vi "Periodic Tasks.vi"(3 "error in":errorcluster) -> ()   [LabVIEW 2020]
doc: "This VI runs in parallel to other tasks. It can contain as many user-defined periodic loops as you need. These can carry out PID or other sorts of timed response."
uses:
  Robot Global Data.vi
  <vilib>/Rock Robotics/WPI/DriverStation/WPI_DriverStationRobotMode2.ctl
  mechanisms.ctl
  <vilib>/Rock Robotics/WPI/ThirdParty/Phoenix-LabVIEW/Motor Controller/Controls/CTRE_Phoenix_MotorControl_ControlMode.ctl
  <vilib>/Rock Robotics/WPI/Solenoid/WPI_SolenoidValue.ctl
  <vilib>/Rock Robotics/WPI/Solenoid/WPI_SolenoidSetEnum.vi
  <vilib>/Rock Robotics/WPI/Solenoid/Deprecated/WPI_SolenoidGetBool.vi
  <vilib>/Rock Robotics/WPI/ThirdParty/REV Robotics/REVLib/Typedef/Spark MAX Control Type.ctl
  <vilib>/Rock Robotics/Network Tables/NT Write Number.vi
  <vilib>/Rock Robotics/Network Tables/NT Write String.vi
  <vilib>/Rock Robotics/WPI/Compressor/WPI_CompressorFeedbackMode.ctl
  <vilib>/Rock Robotics/Network Tables/NT Write Numeric Array.vi
  <vilib>/Rock Robotics/WPI/DriverStation/WPI_DriverStationAllianceInfo.ctl
  <vilib>/Rock Robotics/WPI/Joystick/WPI_JoystickDeviceEnum.ctl
  <vilib>/Rock Robotics/WPI/Joystick/WPI_JoystickDevRef.ctl
  Front Left Output.ctl
  Back Left Outputctl.ctl
  Back Right Output.ctl
  Front Right Output.ctl
panel:
  in  "HIgh Left 2":dbl=-100.0
  in  "High Right 2":dbl=-100.0
  in  "Reset Position":bool
  in  "High Right":dbl=-100.0
  in  "Elevator Dealy":i32=80
  out "Left Pulse Switch":bool
  out "Right Pulse Switch":bool
  in  "HIgh Left":dbl=-100.0
  in  "Low Goal":dbl=10.0
  out "Back Right RPM":dbl
  out "Front Right RPM":dbl
  out "Back Left RPM":dbl
  out "Front Left RPM":dbl
  out "Alliance":T1
  in  "Align 90":bool
  out "Auto Step":dbl
  out "Front Left Drive Position":dbl
  out "Low Pressure":dbl
  in  "Piston Delay":i32=2
  out "Compressor Running":bool
  out "Enabled":bool
  in  "Disable Compressor":bool
  out "High Pressure":dbl(slide) scale=0.0..120.0
  in  "Max Pressure (PSI)":dbl(slide)=120.0 scale=0.0..120.0
  in  "Min Pressure (PSI)":dbl(slide)=100.0 scale=0.0..120.0
  out "Left Color":string
  out "Left Color":u32(colorbox)
  in  "Blue Calibration":cluster{"R":dbl, "G":dbl, "B":dbl}={"R"=0.159091, "G"=0.404537, "B"=0.435606}
  in  "Green Calibration":cluster{"R":dbl, "G":dbl, "B":dbl}={"R"=0.282, "G"=0.513, "B"=0.204}
  in  "Red Calibration":cluster{"R":dbl, "G":dbl, "B":dbl}={"R"=0.583685, "G"=0.333333, "B"=0.082982}
  in  "Yellow Calibration":cluster{"R":dbl, "G":dbl, "B":dbl}={"R"=0.309, "G"=0.524, "B"=0.166}
  in  "Rear Stop":dbl=-410.0
  in  "Front Stop":dbl=-280.0
  out "Right Color Match":string
  out "Right Color":u32(colorbox)
  out "Front Climber Switch":bool
  out "Rear Climber Switch":bool
  out "Claw Piston":bool
  out "Left Intake Piston":bool
  out "Right Intake Piston":bool
  out "Left Shooter":bool
  out "Right Shooter":bool
  out "Front Climber Postion":dbl
  out "Rear Climber Postion":dbl
  out "comp yaw":dbl=98.73633599999974 format="%#.1f"
  out "Linear Acceleration":T2={"LinearAcceleration X"=0.0, "LinearAcceleration Y"=0.002, "LinearAcceleration Z"=0.012}
  in  "Front Left Offset":dbl=589.0
  in  "Front Right Offset":dbl=547.0
  in  "Back Left Offset":dbl=743.0
  in  "Back Right Offset":dbl=1064.0
  out "Left Front Drive Output":T3={"Front Left Velocity"=-0.0, "Front Left Current Angle"=179.67273538762845, "Front Left Position (Raw Sensor Units)"=936}
  out "Back Left Drive Output":T4={"Back Left Back Velocity"=0.0, " Back Left Current Angle"=359.61772051724495, "Back Left Position (Raw Sensor Units)"=790}
  out "Back Right Drive Output":T5={"Back Right Velocity"=0.0, "Back Right Current Angle"=0.24094689976084283, "Back Left Position (Raw Sensor Units)"=126}
  out "Right  Front Drive Output":T6={"Front Right Velocity"=0.0, "Front Right Current Angle"=0.5093765258786789, "Front Right Position (Raw Sensor Units)"=548}
  in  "Joystick Addresses":cluster{"Auxillary":T7, "Driver":T7}
  # "Max RPM 5700"
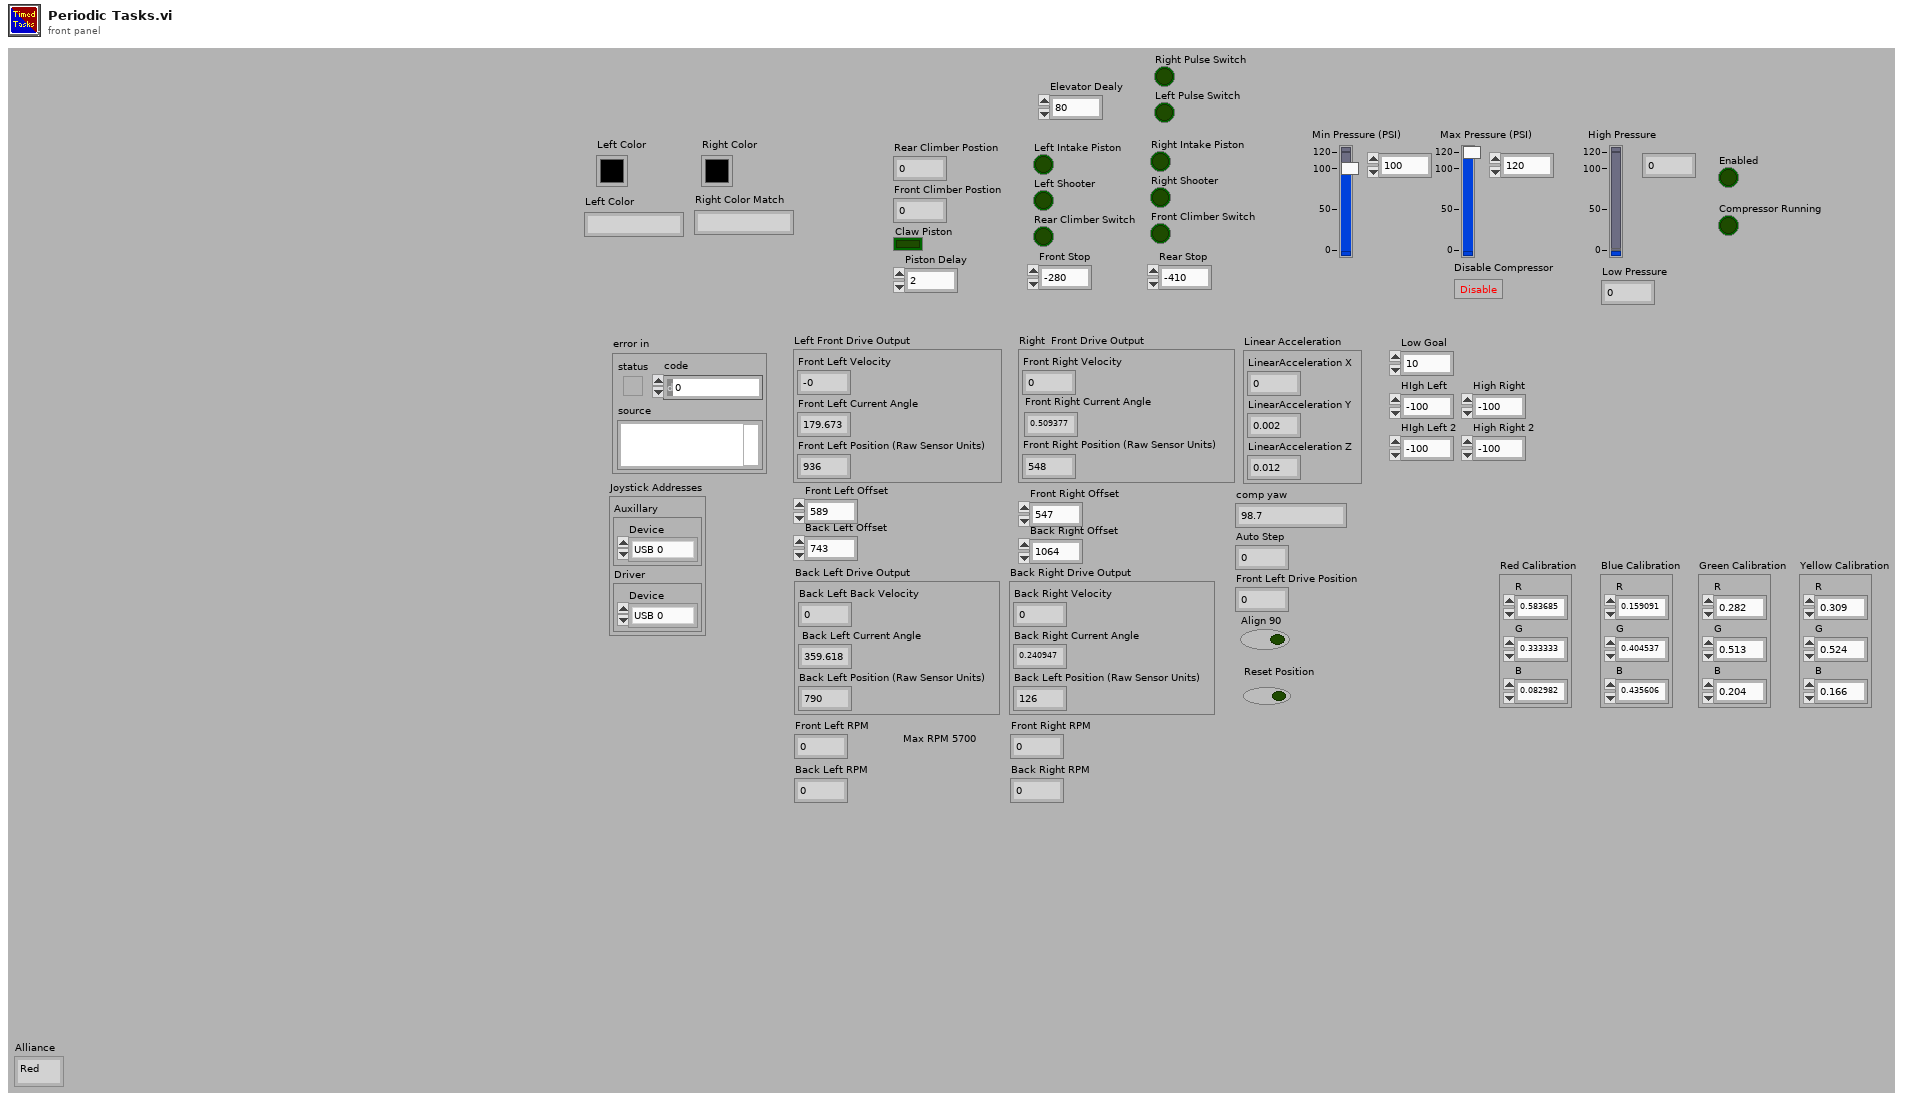
[diagram p1: front panel]
types:
  T1 = typedef "WPI_DriverStationAllianceInfo.ctl" = enum16{"Red", "Blue", "Invalid"}
  T2 = cluster{"LinearAcceleration X":dbl, "LinearAcceleration Y":dbl, "LinearAcceleration Z":dbl}
  T3 = typedef "Front Left Output.ctl" = cluster{"Front Left Velocity":dbl, "Front Left Current Angle":dbl, "Front Left Position (Raw Sensor Units)":i32}
  T4 = typedef "Back Left Outputctl.ctl" = cluster{"Back Left Back Velocity":dbl, " Back Left Current Angle":dbl, "Back Left Position (Raw Sensor Units)":i32}
  T5 = typedef "Back Right Output.ctl" = cluster{"Back Right Velocity":dbl, "Back Right Current Angle":dbl, "Back Left Position (Raw Sensor Units)":i32}
  T6 = typedef "Front Right Output.ctl" = cluster{"Front Right Velocity":dbl, "Front Right Current Angle":dbl, "Front Right Position (Raw Sensor Units)":i32}
  T7 = typedef "WPI_JoystickDevRef.ctl" = cluster{"Device":T8}
  T8 = typedef "WPI_JoystickDeviceEnum.ctl" = enum16{"USB 0", "USB 1", "USB 2", "USB 3", "USB 4", "USB 5"}
  T9 = typedef "WPI_DriverStationRobotMode2.ctl" = enum16{"Autonomous Disabled", "Autonomous Enabled", "Teleop Disabled", "Teleop Enabled", "Disconnected", "Finish", "Test Disabled", "Test Enabled", "Emergency Stopped"}
  T10 = typedef "mechanisms.ctl" = string
  T11 = cluster{"Yaw":dbl, "Roll":dbl, "Pitch":dbl, "Heading":dbl, "Fused Heading":dbl}
  T12 = cluster{"L X Axis":dbl, "L Y Axis":dbl, "LT":dbl, "RT":dbl, "R X Axis":dbl, "R Y Axis":dbl}
  T13 = cluster{"A":bool, "B":bool, "X":bool, "Y":bool, "LB":bool, "RB":bool, "Back":bool, "Start":bool, "Left Stick Push":bool, "Right Stick Push":bool}
  T14 = typedef "Color Sensor V3 DevRef.ctl" = cluster{"I2CDevRef":T15}
  T15 = typedef "WPI_I2CDevRef.ctl" = cluster{"DevStatus":errorcluster, "Device Address":u8, "Handle":i32, "I2C Bus":T16}
  T16 = typedef "i2c_bus.ctl" = enum16{"I2C On-Board", "I2C MXP", "Invalid"}
  T17 = typedef "WPI_MotorControlDeviceRef.ctl" = cluster{"DeviceStatus":errorcluster, "Type":T18, "PWM":cluster{"PWM Channel":T19, "DeadBand":T20}, "CAN":cluster{"Device Number":u8, "SetOutput VI Ref":variant, "GetOutput VI Ref":variant, "Enable VI Ref":variant, "Disable VI Ref":variant, "Data":variant}, "Invert":bool, "DIO PWM":cluster{"PWM \"Enable\" Channel":T19, "DIOChannel":T21, "PWM Rate":dbl}}
  T18 = typedef "WPI_MotorControlType.ctl" = enum16{"PWM", "CAN", "DIO PWM"}
  T19 = typedef "FPGA_DIOPWMChannel.ctl" = enum8{"PWM 0", "PWM 1", "PWM 2", "PWM 3", "PWM 4", "PWM 5", "PWM 6", "PWM 7", "PWM 8", "PWM 9", "PWM MXP 0", "PWM MXP 1", "PWM MXP 2", "PWM MXP 3", "PWM MXP 4", "PWM MXP 5", "PWM MXP 6", "PWM MXP 7", "PWM MXP 8", "PWM MXP 9", "Invalid"}
  T20 = typedef "WPI_PWMDeadband.ctl" = cluster{"Name":string, "maxPositivePwm":i32, "minPositivePwm":i32, "centerPwm":i32, "maxNegativePwm":i32, "minNegativePwm":i32, "angularRange":u16}
  T21 = typedef "FPGA_DIOChannel.ctl" = enum8{"DIO 0", "DIO 1", "DIO 2", "DIO 3", "DIO 4", "DIO 5", "DIO 6", "DIO 7", "DIO 8", "DIO 9", "DIO MXP 0", "DIO MXP 1", "DIO MXP 2", "DIO MXP 3", "DIO MXP 4", "DIO MXP 5", "DIO MXP 6", "DIO MXP 7", "DIO MXP 8", "DIO MXP 9", "DIO MXP 10", "DIO MXP 11", "DIO MXP 12", "DIO MXP 13", "DIO MXP 14", "DIO MXP 15", "SPI Port CS1", "SPI Port CS2", "SPI Port CS3", "SPI Port MISO", "SPI Port MOSI", "Invalid"}
  T22 = typedef "WPI_SolenoidValue.ctl" = enum16{"Off", "On", "Forward", "Reverse"}
  T23 = typedef "WPI_DigitalInputDevRef.ctl" = cluster{"DevStatus":errorcluster, "DIO Channel":T21}
  T24 = typedef "WPI_SolenoidDevRef.ctl" = cluster{"DevStatus":errorcluster, "Pneumatics Control Module":u8, "Forward Solenoid Channel":T25, "Reverse Solenoid Channel":T25}
  T25 = typedef "WPI_SolenoidChannel.ctl" = enum8{"Solenoid 0", "Solenoid 1", "Solenoid 2", "Solenoid 3", "Solenoid 4", "Solenoid 5", "Solenoid 6", "Solenoid 7", "Solenoid 8", "Solenoid 9", "Solenoid 10", "Solenoid 11", "Solenoid 12", "Solenoid 13", "Solenoid 14", "Solenoid 15", "Invalid"}
  T26 = typedef "CTRE_Phoenix_MotorControl_ControlMode.ctl" = u16
  T27 = typedef "WPI_CompressorFeedbackMode.ctl" = enum16{"Analog Only", "Digital Only", "Hybrid"}
  T28 = cluster{"Feedback Sensor":T27, "Max Pressure (PSI)":dbl, "Min Pressure (PSI)":dbl}
  T29 = typedef "WPI_CompressorDevRef.ctl" = cluster{"DevStatus":errorcluster, "Pneumatics Control Module":u8}
  T30 = cluster{"Pressure 0 (psi)":dbl, "Pressure 1 (psi)":dbl}
  T31 = typedef "Direction Commands.ctl" = cluster{"Lateral - X":dbl, "Longitudinal - Y":dbl, "Rotational - Z":dbl}
  T32 = typedef "Drive Comands.ctl" = cluster{"Align Steer Motors":bool, "Brake":bool, "Coast":bool, "Autonomous":bool}
  T33 = typedef "Spark MAX Control Type.ctl" = enum16{"Percent VBus", "Voltage", "Velocity", "Position", "Smart Motion", "Current", "Smart Velocity"}
  T34 = typedef "WPI_SwitchDevRef.ctl" = cluster{"DevStatus":errorcluster, "DIO Channel":T21, "CntIndex":T35, "Normally Closed":bool}
  T35 = typedef "FPGA_CounterCtrSystemIndex.ctl" = enum8{"Ctr 0", "Ctr 1", "Ctr 2", "Ctr 3", "Ctr 4", "Ctr 5", "Ctr 6", "Ctr 7", "Invalid"}
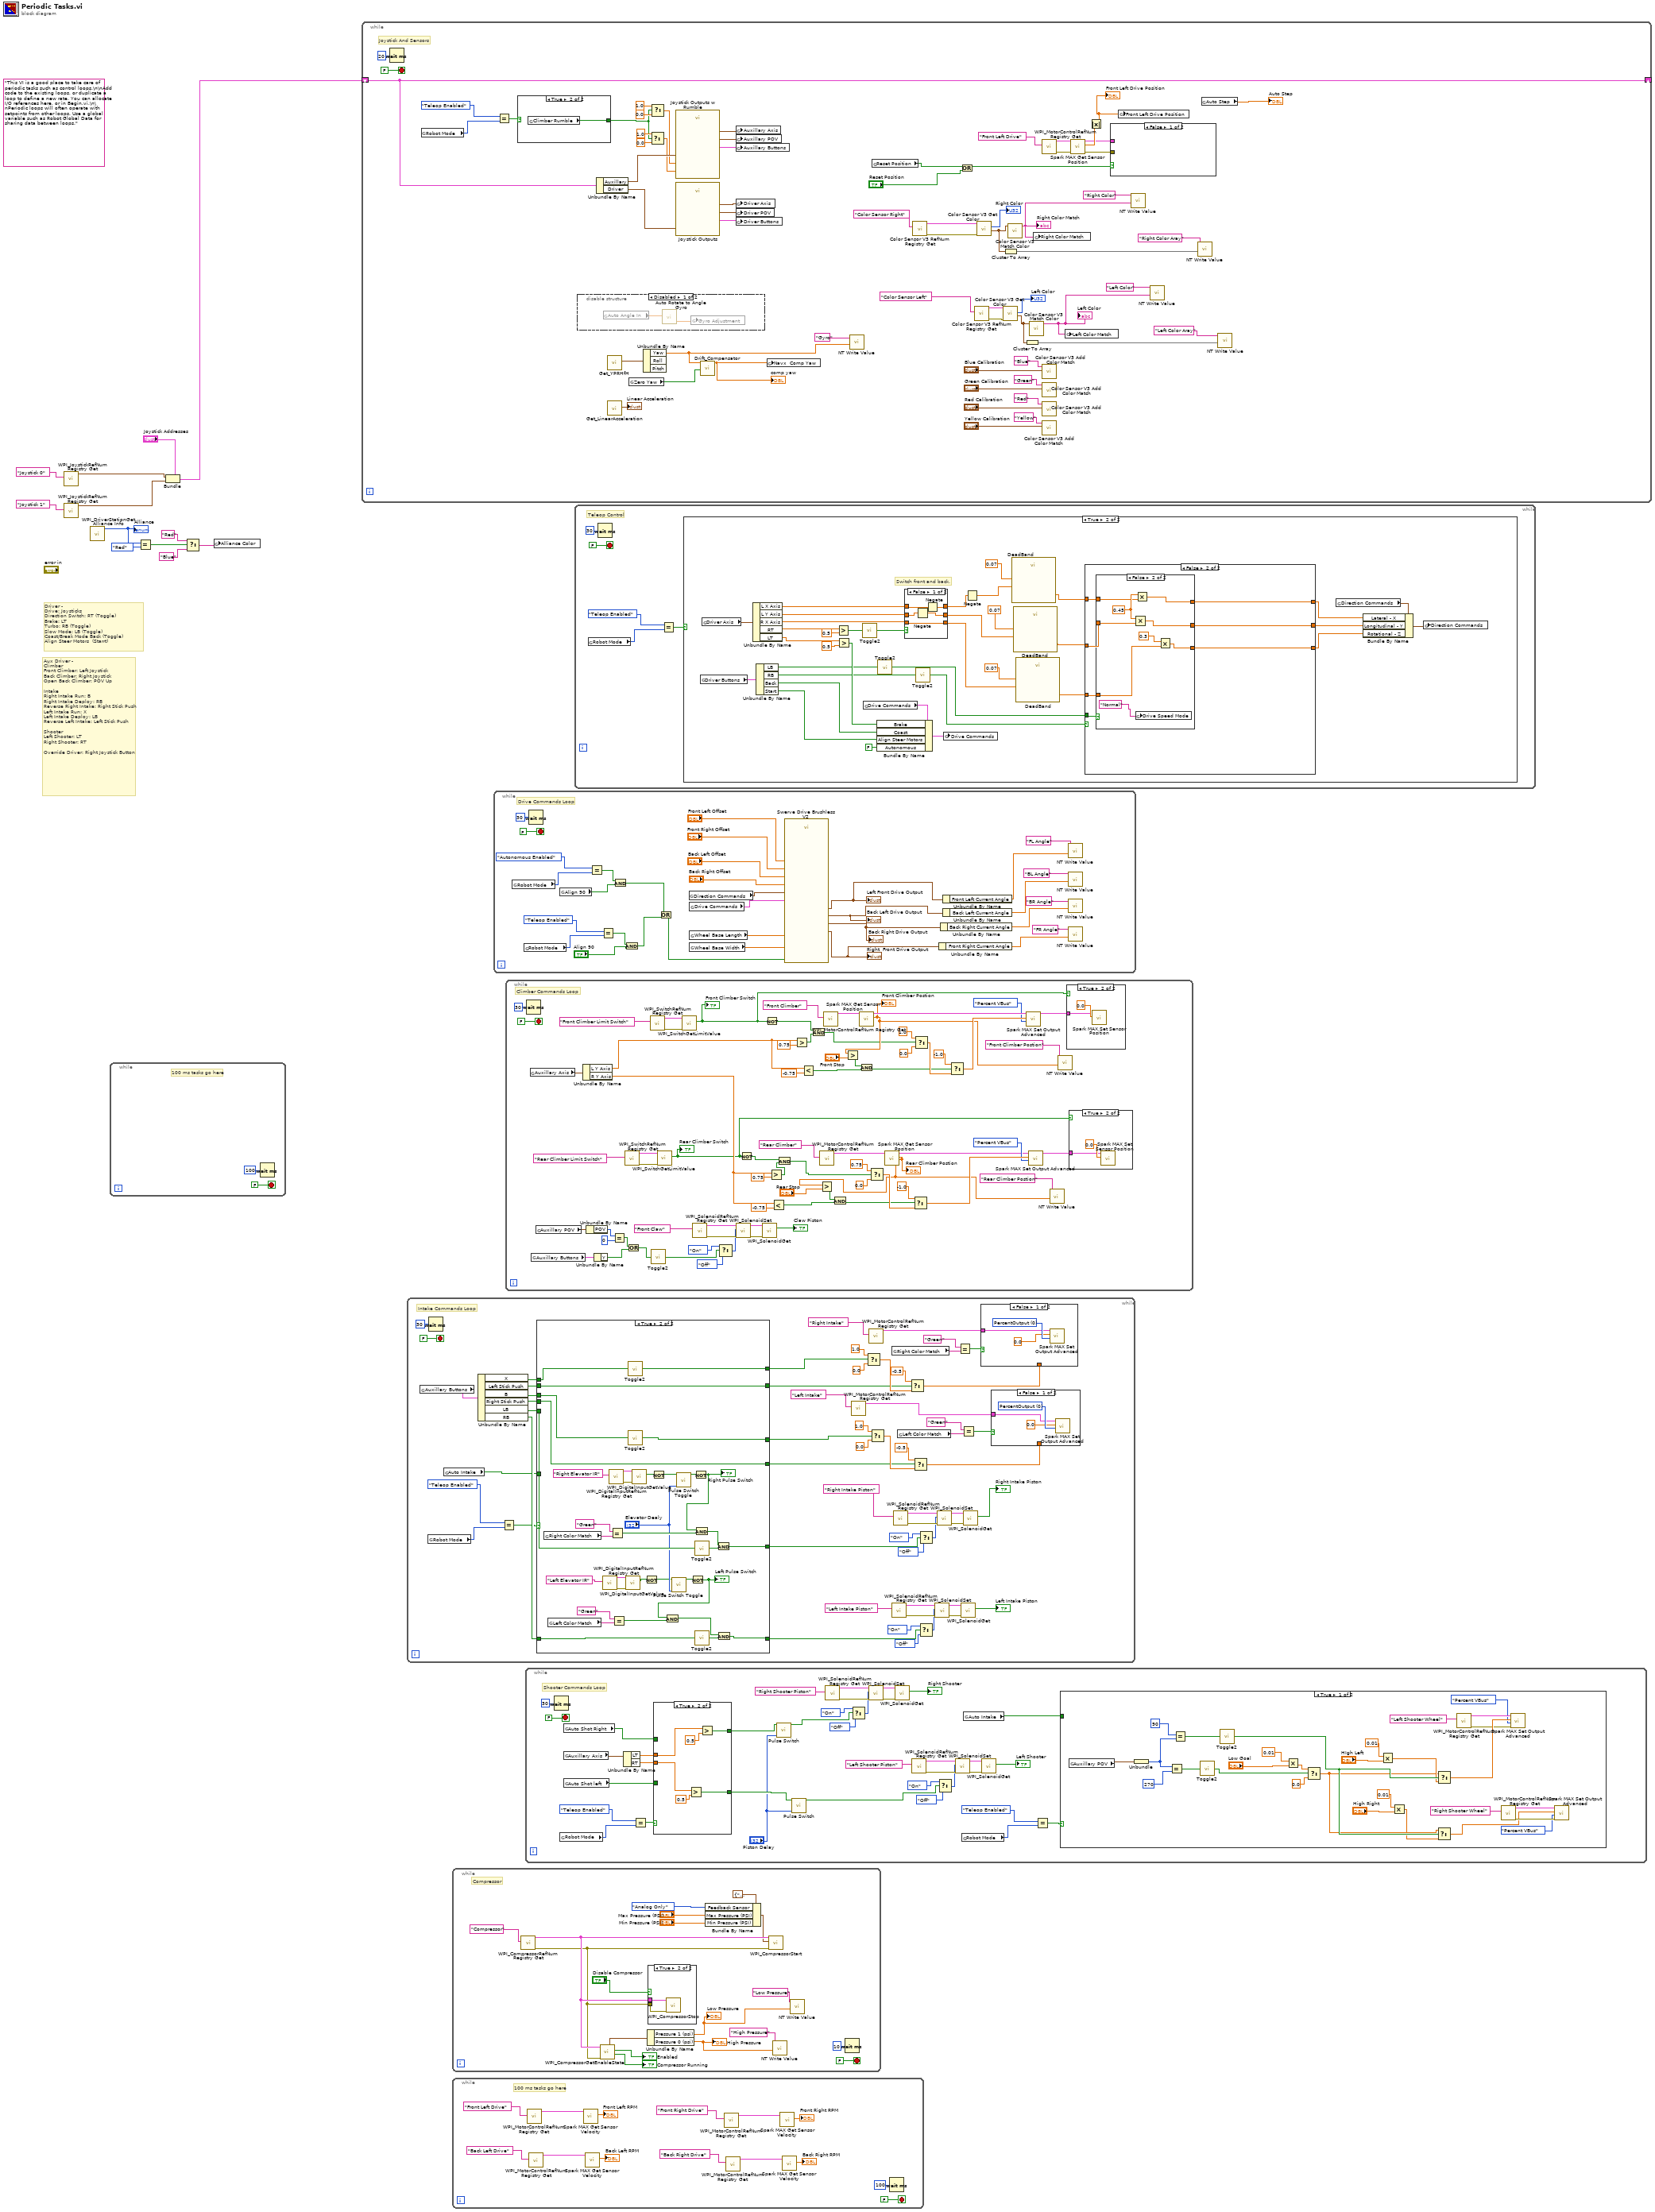
[diagram p0: block diagram]
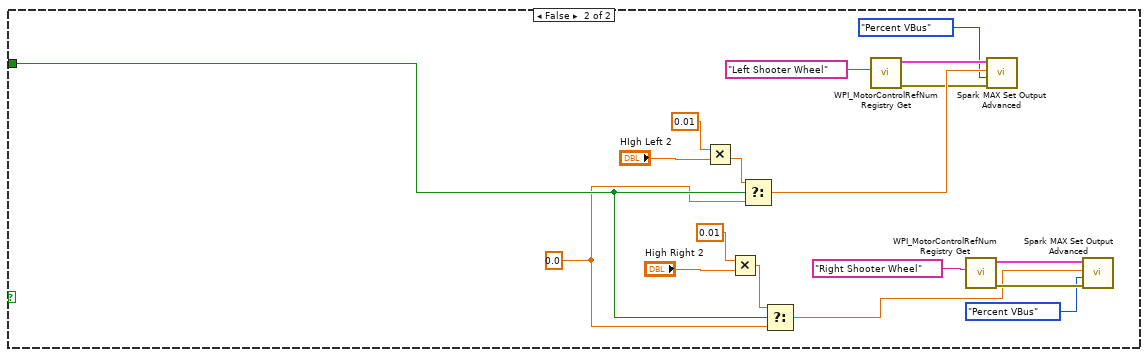
[diagram p3: hidden frame]
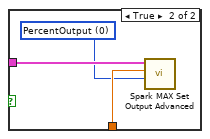
[diagram p5: hidden frame]
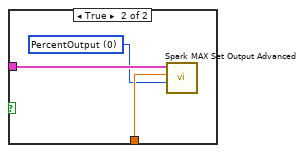
[diagram p6: hidden frame]
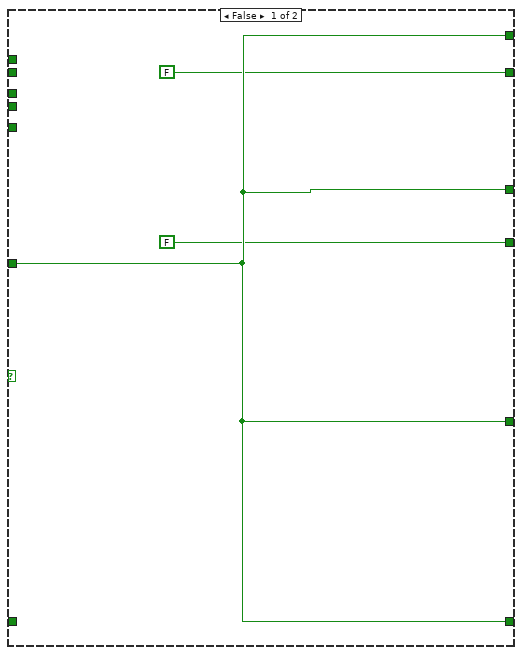
[diagram p7: hidden frame]
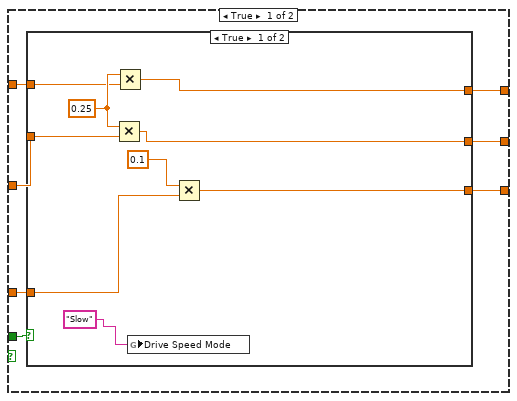
[diagram p11: hidden frame]
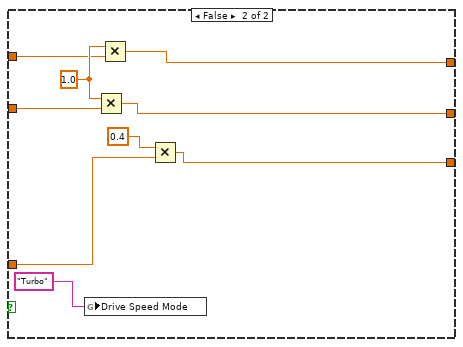
[diagram p12: hidden frame]
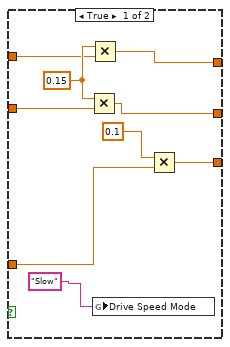
[diagram p13: hidden frame]
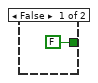
[diagram p15: hidden frame]
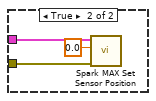
[diagram p17: hidden frame]
diagram:
  (unwired) "This VI is a good place to take care of periodic tasks such as control loops.\n\nAdd code to the existing loops, or duplicate a loop to define a new rate. You can allocate I/O references here, or in Begin.vi.\n\nPeriodic loops will often operate with setpoints from other loops. Use a global variable such as Robot Global Data for sharing data between loops."
  # "Aux Driver - \nClimber\nFront Climber: Left Joystick\nBack Climber: Right Joystick\nOpen Back Climber: POV Up\n\nIntake\nRight Intake Run: B\nRight Intake Deploy: RB\nReverse Right Intake: Right Stick Push\nLeft Intake Run: X\nLeft Intake Deploy: LB\nReverse Left Intake: Left Stick Push\n\nShooter\nLeft Shooter: LT\nRight Shooter: RT\n\nOverride Driver: Right Joystick Button"
  # "Driver - \nDrive: Joysticks\nDirection Switch: RT (Toggle)\nBrake: LT \nTurbo: RB (Toggle) \nSlow Mode: LB (Toggle) \nCoast/Break Mode Back (Toggle)\nAlign Steer Motors  (Starrt)"
  n1 = call <vilib>:"WPI_JoystickRefNum Registry Get.vi"("refnum name"="Joystick 0" ("Joystick Reference")) -> ("JoystickDevRef"=w10:T7)  [unwired: 9 in, 1 out]
  n2 = call <vilib>:"WPI_JoystickRefNum Registry Get.vi"("refnum name"="Joystick 1" ("Joystick Reference")) -> ("JoystickDevRef"=w9:T7)  [unwired: 9 in, 1 out]
  n3 = call <vilib>:"WPI_DriverStationGet Alliance Info.vi"() -> ("Alliance"=w6:T1)  [unwired: 6 in, 5 out]
  "Alliance" <- w6
  n4 = while {
    stop <- FALSE stop-if-true
    # "100 ms tasks go here"
    n5 = Wait (ms)(milliseconds to wait=u32 100) -> ()  [unwired: 1 out]
  }
  n6 = Equal?(x=w6, y=WPI_DriverStationAllianceInfo."Red") -> (x = y?=w4:bool)
  n7 = Bundle(cluster="Joystick Addresses", "Auxillary"=w10, "Driver"=w9) -> (w8:cluster{"Auxillary":T7, "Driver":T7})
  n8 = Select(t="Red" ("Right Color Match 2"), s=w4, f="Blue" ("Right Color Match 2")) -> (s? t:f=w1:string)
  n9 = global write "Robot Global Data.vi" "Alliance Color"(w1) -> ()
  n10 = while {
    shift-right: [w76] -> _
    shift-left: w8 -> [w76]
    stop <- FALSE stop-if-true
    # "Joystick And Sensors"
    n11 = Wait (ms)(milliseconds to wait=u32 20) -> ()  [unwired: 1 out]
    n12 = global read "Robot Global Data.vi" "Robot Mode"() -> (w17:T9)
    n13 = Equal?(x=WPI_DriverStationRobotMode2."Teleop Enabled", y=w17) -> (x = y?=w15:bool)
    n14 = case shown="True" w15 {
      tunnel: [FALSE ("Climber Rumble") w80] -> w20
      frame False {
      }
      frame True {
        n15 = global read "Robot Global Data.vi" "Climber Rumble"() -> (w80:bool)
      }
    }
    n16 = disable-structure shown="Disabled" {
      frame Disabled {
        n17 = global read "Robot Global Data.vi" "Auto Angle In"() -> (w82:dbl)
        n18 = call "Auto Rotate to Angle Gyro.vi"("Drive to Angle"=w82) -> ("Rotational Adjustment"=w81:dbl)  [unwired: 2 in]
        n19 = global write "Robot Global Data.vi" "Gyro Adjustment"(w81) -> ()
      }
      frame Enabled {
      }
    }
    n20 = Unbundle By Name(w76) -> ("Auxillary"=w75:T7, "Driver"=w74:T7)
    n21 = call <vilib>:"Get_YPRHfH.vi"() -> ("YRPHfH"=w63:T11)  [unwired: 11 in]
    n22 = call <vilib>:"Get_LinearAcceleration.vi"() -> ("Linear Acceleration"=→"Linear Acceleration":T2)  [unwired: 11 in]
    n23 = global read "Robot Global Data.vi" "Zero Yaw"() -> (w62:bool)
    n24 = Unbundle By Name(w63) -> ("Yaw"=w61:dbl)  [unwired: 2 out]
    n25 = Select(t=1.0, s=w20, f=0.0) -> (s? t:f=w23:dbl)
    n26 = Select(t=1.0, s=w20, f=0.0) -> (s? t:f=w28:dbl)
    n27 = call "Joystick Outputs w Rumble.vi"("Right Rumble"=w23, "Left Rumble"=w28, "JoystickDevRef"=w75) -> ("POV"=w72:cluster{"POV":i16}, "Axis"=w73:T12, "Buttons"=w71:T13)
    n28 = call "Joystick Outputs.vi"("JoystickDevRef"=w74) -> ("Buttons"=w68:T13, "Axis"=w70:T12, "POV"=w69:cluster{"POV":i16})
    n29 = call <vilib>:"Drift_Compensator.vi"("Zero Yaw"=w62, "Raw Yaw"=w61) -> ("comp yaw"=w60:dbl)  [unwired: 9 in]
    "comp yaw" <- w60
    n30 = global write "Robot Global Data.vi" "Auxillary Axis"(w73) -> ()
    n31 = global write "Robot Global Data.vi" "Auxillary POV"(w72) -> ()
    n32 = global write "Robot Global Data.vi" "Auxillary Buttons"(w71) -> ()
    n33 = global write "Robot Global Data.vi" "Driver Axis"(w70) -> ()
    n34 = global write "Robot Global Data.vi" "Driver POV"(w69) -> ()
    n35 = global write "Robot Global Data.vi" "Driver Buttons"(w68) -> ()
    n36 = global write "Robot Global Data.vi" "Navx  Comp Yaw"(w60) -> ()
    n37 = call-poly <vilib>:"NT Write Value.vi"("Numeric"=w61, "Name"="Gyro") -> ()  [unwired: 9 in, 1 out]
    n38 = global read "Robot Global Data.vi" "Reset Position"() -> (w31:bool)
    n39 = call <vilib>:"Color Sensor V3 RefNum Registry Get.vi"("refnum name"=T10 "Color Sensor Right" ("Mechanism")) -> ("error out"=w56:errorcluster, "ColorSensorDevRef"=w55:T14)  [unwired: 9 in]
    n40 = Or(x=w31, y="Reset Position") -> (x .or. y?=w19:bool)
    n41 = call <vilib>:"Color Sensor V3 RefNum Registry Get.vi"("refnum name"=T10 "Color Sensor Left" ("Mechanism")) -> ("error out"=w52:errorcluster, "ColorSensorDevRef"=w53:T14)  [unwired: 9 in]
    n42 = call <vilib>:"Color Sensor V3 Get Color.vi"("error in (no error)"=w56, "ColorSensorDevRef"=w55) -> ("Normalized Color"=w40:cluster{"R":dbl, "G":dbl, "B":dbl}, "Color"=→"Right Color":u32)  [unwired: 6 in, 2 out]
    n43 = call <vilib>:"Color Sensor V3 Get Color.vi"("error in (no error)"=w52, "ColorSensorDevRef"=w53) -> ("Normalized Color"=w36:cluster{"R":dbl, "G":dbl, "B":dbl}, "Color"=→"Left Color":u32)  [unwired: 6 in, 2 out]
    n44 = Cluster To Array(cluster=w40) -> (array=w39:dbl[])
    n45 = call <vilib>:"Color Sensor V3 Match Color.vi"("Measured Color"=w40) -> ("Matched Color Name"=w21:string)  [unwired: 8 in, 2 out]
    "Right Color Match" <- w21
    n46 = Cluster To Array(cluster=w36) -> (array=w35:dbl[])
    n47 = call <vilib>:"Color Sensor V3 Match Color.vi"("Measured Color"=w36) -> ("Matched Color Name"=w22:string)  [unwired: 8 in, 2 out]
    "Left Color" <- w22
    n48 = global write "Robot Global Data.vi" "Right Color Match"(w21) -> ()
    n49 = call <vilib>:"WPI_MotorControlRefNum Registry Get.vi"("refnum name"="Front Left Drive" ("Motor References")) -> ("error out"=w65:errorcluster, "RobotDriveDevRef"=w66:T17)  [unwired: 9 in]
    n50 = call <vilib>:"Color Sensor V3 Add Color Match.vi"("Color"="Blue Calibration", "Name"="Blue") -> ()  [unwired: 10 in]
    n51 = call <vilib>:"Color Sensor V3 Add Color Match.vi"("Color"="Green Calibration", "Name"="Green") -> ()  [unwired: 10 in]
    n52 = call <vilib>:"Color Sensor V3 Add Color Match.vi"("Color"="Red Calibration", "Name"="Red") -> ()  [unwired: 10 in]
    n53 = call <vilib>:"Color Sensor V3 Add Color Match.vi"("Color"="Yellow Calibration", "Name"="Yellow") -> ()  [unwired: 10 in]
    n54 = global write "Robot Global Data.vi" "Left Color Match"(w22) -> ()
    n55 = call <vilib>:"Spark MAX Get Sensor Position.vi"("error in (no error)"=w65, "MotorControlDevRef in"=w66) -> ("error out"=w32:errorcluster, "Sensor Position"=w34:dbl, "MotorControlDevRef out"=w33:T17)  [unwired: 6 in, 1 out]
    n56 = Absolute Value(x=w34) -> (abs(x)=w29:dbl)
    "Front Left Drive Position" <- w29
    n57 = case shown="False" w19 {
      tunnel: w33 -> [_ w85]
      tunnel: w32 -> [_ w84]
      frame False {
      }
      frame True {
        n58 = call <vilib>:"Spark MAX Set Sensor Position.vi"("error in"=w84, "Position"=0.0, "MotorControlDeviceRef"=w85) -> ()  [unwired: 7 in, 2 out]
      }
    }
    n59 = global write "Robot Global Data.vi" "Front Left Drive Position"(w29) -> ()
    n60 = call-poly <vilib>:"NT Write Value.vi"("String"=w21, "Name"="Right Color") -> ()  [unwired: 9 in, 1 out]
    n61 = call-poly <vilib>:"NT Write Value.vi"("String"=w22, "Name"="Left Color") -> ()  [unwired: 9 in, 1 out]
    n62 = call-poly <vilib>:"NT Write Value.vi"("Numeric Array"=w39, "Name"="Right Color Aray") -> ()  [unwired: 9 in, 1 out]
    n63 = global read "Robot Global Data.vi" "Auto Step"() -> (→"Auto Step":dbl)
    n64 = call-poly <vilib>:"NT Write Value.vi"("Numeric Array"=w35, "Name"="Left Color Aray") -> ()  [unwired: 9 in, 1 out]
  }
  n65 = while {
    stop <- FALSE stop-if-true
    # "Intake Commands Loop"
    n66 = global read "Robot Global Data.vi" "Auxillary Buttons"() -> (w140:T13)
    n67 = global read "Robot Global Data.vi" "Robot Mode"() -> (w99:T9)
    n68 = Wait (ms)(milliseconds to wait=u32 30) -> ()  [unwired: 1 out]
    n69 = global read "Robot Global Data.vi" "Auto Intake"() -> (w96:bool)
    n70 = Unbundle By Name(w140) -> ("X"=w124:bool, "Left Stick Push"=w93:bool, "B"=w125:bool, "Right Stick Push"=w91:bool, "LB"=w102:bool, "RB"=w101:bool)
    n71 = Equal?(x=WPI_DriverStationRobotMode2."Teleop Enabled", y=w99) -> (x = y?=w97:bool)
    n72 = case shown="True" w97 {
      tunnel: w125 -> [_ w192]
      tunnel: w124 -> [_ w191]
      tunnel: [w157 w190] -> w123
      tunnel: [w157 w180] -> w105
      tunnel: [w157 w177] -> w104
      tunnel: w102 -> [_ w189]
      tunnel: w101 -> [_ w188]
      tunnel: [w157 w187] -> w100
      tunnel: w96 -> [w157 _]
      tunnel: w93 -> [_ w186]
      tunnel: [FALSE ("Left Stick Push") w186] -> w92
      tunnel: w91 -> [_ w185]
      tunnel: [FALSE ("Right Stick Push") w185] -> w90
      frame False {
      }
      frame True {
        n73 = global read "Robot Global Data.vi" "Right Color Match"() -> (w183:string)
        n74 = global read "Robot Global Data.vi" "Left Color Match"() -> (w182:string)
        n75 = call <vilib>:"WPI_DigitalInputRefNum Registry Get.vi"("refnum name"=T10 "Left Elevator IR" ("Mechanisms")) -> ("error out"=w173:errorcluster, "DigitalInputDevRef"=w172:T23)  [unwired: 9 in]
        n76 = call <vilib>:"WPI_DigitalInputRefNum Registry Get.vi"("refnum name"=T10 "Right Elevator IR" ("Mechanisms")) -> ("error out"=w175:errorcluster, "DigitalInputDevRef"=w174:T23)  [unwired: 9 in]
        n77 = Equal?(x="Green", y=w183) -> (x = y?=w169:bool)
        n78 = Equal?(x="Green", y=w182) -> (x = y?=w167:bool)
        n79 = call <vilib>:"WPI_DigitalInputGetValue.vi"("error in (no error)"=w173, "DigitalInputDevRef"=w172) -> ("Value"=w170:bool)  [unwired: 7 in, 2 out]
        n80 = call "Toggle2.vi"("In 2"=w191) -> ("Out 2"=w187:bool)
        n81 = call "Toggle2.vi"("In 2"=w192) -> ("Out 2"=w190:bool)
        n82 = call <vilib>:"WPI_DigitalInputGetValue.vi"("error in (no error)"=w175, "DigitalInputDevRef"=w174) -> ("Value"=w166:bool)  [unwired: 7 in, 2 out]
        n83 = Not(x=w170) -> (.not. x?=w162:bool)
        n84 = Not(x=w166) -> (.not. x?=w163:bool)
        n85 = call "Pulse Switch Toggle.vi"("Input Switch"=w162, "Time/Loop Time"="Elevator Dealy") -> ("Pulse Switch"=w168:bool)  [unwired: 7 in, 1 out]
        n86 = call "Pulse Switch Toggle.vi"("Input Switch"=w163, "Time/Loop Time"="Elevator Dealy") -> ("Pulse Switch"=w165:bool)  [unwired: 7 in, 1 out]
        n87 = Not(x=w168) -> (.not. x?=w160:bool)
        "Left Pulse Switch" <- w160
        n88 = And(x=w160, y=w167) -> (x .and. y?=w161:bool)
        n89 = Not(x=w165) -> (.not. x?=w158:bool)
        "Right Pulse Switch" <- w158
        n90 = call "Toggle2.vi"("In 2"=w189) -> ("Out 2"=w179:bool)
        n91 = call "Toggle2.vi"("In 2"=w188) -> ("Out 2"=w178:bool)
        n92 = And(x=w158, y=w169) -> (x .and. y?=w159:bool)
        n93 = And(x=w159, y=w179) -> (x .and. y?=w180:bool)
        n94 = And(x=w161, y=w178) -> (x .and. y?=w177:bool)
      }
    }
    n95 = call <vilib>:"WPI_MotorControlRefNum Registry Get.vi"("refnum name"=T10 "Left Intake" ("Mechanism")) -> ("RobotDriveDevRef"=w133:T17)  [unwired: 9 in, 1 out]
    n96 = Select(t=1.0, s=w100, f=0.0) -> (s? t:f=w131:dbl)
    n97 = call <vilib>:"WPI_MotorControlRefNum Registry Get.vi"("refnum name"=T10 "Right Intake" ("Mechanism")) -> ("RobotDriveDevRef"=w126:T17)  [unwired: 9 in, 1 out]
    n98 = Select(t=1.0, s=w123, f=0.0) -> (s? t:f=w138:dbl)
    n99 = call <vilib>:"WPI_SolenoidRefNum Registry Get.vi"("refnum name"=T10 "Left Intake Piston" ("Mechanism")) -> ("error out"=w113:errorcluster, "SolenoidDevRef"=w112:T24)  [unwired: 9 in]
    n100 = global read "Robot Global Data.vi" "Right Color Match"() -> (w95:string)
    n101 = call <vilib>:"WPI_SolenoidRefNum Registry Get.vi"("refnum name"=T10 "Right Intake Piston" ("Mechanism")) -> ("error out"=w122:errorcluster, "SolenoidDevRef"=w121:T24)  [unwired: 9 in]
    n102 = global read "Robot Global Data.vi" "Left Color Match"() -> (w88:string)
    n103 = Select(t=-0.5, s=w92, f=w131) -> (s? t:f=w128:dbl)
    n104 = Select(t=-0.5, s=w90, f=w138) -> (s? t:f=w135:dbl)
    n105 = Select(t=WPI_SolenoidValue."On" ("Value"), s=w104, f=WPI_SolenoidValue."Off" ("Value")) -> (s? t:f=w109:T22)
    n106 = Select(t=WPI_SolenoidValue."On" ("Value"), s=w105, f=WPI_SolenoidValue."Off" ("Value")) -> (s? t:f=w118:T22)
    n107 = call-poly <vilib>:"WPI_SolenoidSet.vi"("error in (no error)"=w113, "Value"=w109, "SolenoidDevRef"=w112) -> ("error out"=w110:errorcluster, "SolenoidDevRef"=w111:T24)  [unwired: 7 in]
    n108 = call-poly <vilib>:"WPI_SolenoidSet.vi"("error in (no error)"=w122, "Value"=w118, "SolenoidDevRef"=w121) -> ("error out"=w119:errorcluster, "SolenoidDevRef"=w120:T24)  [unwired: 7 in]
    n109 = Equal?(x="Green", y=w95) -> (x = y?=w87:bool)
    n110 = call-poly <vilib>:"WPI_SolenoidGet.vi"("error in (no error)"=w110, "SolenoidDevRef"=w111) -> ("Value"=→"Left Intake Piston":bool)  [unwired: 7 in, 2 out]
    n111 = Equal?(x="Green", y=w88) -> (x = y?=w86:bool)
    n112 = call-poly <vilib>:"WPI_SolenoidGet.vi"("error in (no error)"=w119, "SolenoidDevRef"=w120) -> ("Value"=→"Right Intake Piston":bool)  [unwired: 7 in, 2 out]
    n113 = case shown="False" w87 {
      tunnel: w128 -> [_ w154]
      tunnel: w126 -> [w149 w153]
      frame False {
        w151 = T26 0 items=["PercentOutput"=0, "Position"=1, "Velocity"=2, "Current"=3, "Follower"=5, "MotionProfile"=6, "MotionMagic"=7, "MotionMagicArc"=8, "MotionProfileArc"=10, "Disabled"=15] ("Control Mode")
        n114 = call <vilib>:"Spark MAX Set Output Advanced.vi"("Control Mode"=w151, "Setpoint"=0.0, "MotorControlDevRef"=w149) -> ()  [unwired: 7 in, 2 out]
      }
      frame True {
        w152 = T26 0 items=["PercentOutput"=0, "Position"=1, "Velocity"=2, "Current"=3, "Follower"=5, "MotionProfile"=6, "MotionMagic"=7, "MotionMagicArc"=8, "MotionProfileArc"=10, "Disabled"=15] ("Control Mode")
        n115 = call <vilib>:"Spark MAX Set Output Advanced.vi"("Control Mode"=w152, "Setpoint"=w154, "MotorControlDevRef"=w153) -> ()  [unwired: 7 in, 2 out]
      }
    }
    n116 = case shown="False" w86 {
      tunnel: w135 -> [_ w148]
      tunnel: w133 -> [w143 w147]
      frame False {
        w145 = T26 0 items=["PercentOutput"=0, "Position"=1, "Velocity"=2, "Current"=3, "Follower"=5, "MotionProfile"=6, "MotionMagic"=7, "MotionMagicArc"=8, "MotionProfileArc"=10, "Disabled"=15] ("Control Mode")
        n117 = call <vilib>:"Spark MAX Set Output Advanced.vi"("Control Mode"=w145, "Setpoint"=0.0, "MotorControlDevRef"=w143) -> ()  [unwired: 7 in, 2 out]
      }
      frame True {
        w146 = T26 0 items=["PercentOutput"=0, "Position"=1, "Velocity"=2, "Current"=3, "Follower"=5, "MotionProfile"=6, "MotionMagic"=7, "MotionMagicArc"=8, "MotionProfileArc"=10, "Disabled"=15] ("Control Mode")
        n118 = call <vilib>:"Spark MAX Set Output Advanced.vi"("Control Mode"=w146, "Setpoint"=w148, "MotorControlDevRef"=w147) -> ()  [unwired: 7 in, 2 out]
      }
    }
  }
  n119 = while {
    stop <- FALSE stop-if-true
    # "Compressor"
    n120 = call <vilib>:"WPI_CompressorRefNum Registry Get.vi"("refnum name"="Compressor") -> ("error out"=w201:errorcluster, "CompressorDevRef"=w202:T29)  [unwired: 9 in]
    n121 = call <vilib>:"WPI_CompressorGetEnableState.vi"("error in (no error)"=w201, "CompressorDevRef"=w202) -> ("Compressor Running"=→"Compressor Running":bool, "Enabled"=→"Enabled":bool, "Pressure Sensors"=w206:T30)  [unwired: 3 in, 4 out]
    n122 = Unbundle By Name(w206) -> ("Pressure 1 (psi)"=w193:dbl, "Pressure 0 (psi)"=w200:dbl)
    "High Pressure" <- w200
    "Low Pressure" <- w193
    n123 = case shown="True" "Disable Compressor" {
      tunnel: w201 -> [_ w212]
      tunnel: w202 -> [_ w211]
      frame False {
      }
      frame True {
        n124 = call <vilib>:"WPI_CompressorStop.vi"("error in (no error)"=w212, "CompressorDevRef"=w211) -> ()  [unwired: 8 in, 2 out]
      }
    }
    n125 = Bundle By Name(cluster=T28 {"Feedback Sensor"=enum."Digital Only", "Max Pressure (PSI)"=0.0, "Min Pressure (PSI)"=0.0} ("Feedback Configuration"), "Feedback Sensor"=WPI_CompressorFeedbackMode."Analog Only", "Max Pressure (PSI)"="Max Pressure (PSI)", "Min Pressure (PSI)"="Min Pressure (PSI)") -> (w197:T28)
    n126 = call <vilib>:"WPI_CompressorStart.vi"("error in (no error)"=w201, "Feedback Configuration"=w197, "CompressorDevRef"=w202) -> ()  [unwired: 7 in, 2 out]
    n127 = call-poly <vilib>:"NT Write Value.vi"("Numeric"=w200, "Name"="High Pressure") -> ()  [unwired: 9 in, 1 out]
    n128 = call-poly <vilib>:"NT Write Value.vi"("Numeric"=w193, "Name"="Low Pressure") -> ()  [unwired: 9 in, 1 out]
    n129 = Wait (ms)(milliseconds to wait=u32 10) -> ()  [unwired: 1 out]
  }
  n130 = while {
    stop <- FALSE stop-if-true
    # "100 ms tasks go here"
    n131 = call <vilib>:"WPI_MotorControlRefNum Registry Get.vi"("refnum name"="Front Left Drive" ("Motor References")) -> ("RobotDriveDevRef"=w224:T17)  [unwired: 9 in, 1 out]
    n132 = call <vilib>:"WPI_MotorControlRefNum Registry Get.vi"("refnum name"="Back Left Drive" ("Motor References")) -> ("RobotDriveDevRef"=w221:T17)  [unwired: 9 in, 1 out]
    n133 = call <vilib>:"Spark MAX Get Sensor Velocity.vi"("MotorControlDevRef in"=w224) -> ("Sensor Velocity"=→"Front Left RPM":dbl)  [unwired: 7 in, 3 out]
    n134 = call <vilib>:"Spark MAX Get Sensor Velocity.vi"("MotorControlDevRef in"=w221) -> ("Sensor Velocity"=→"Back Left RPM":dbl)  [unwired: 7 in, 3 out]
    n135 = call <vilib>:"WPI_MotorControlRefNum Registry Get.vi"("refnum name"="Front Right Drive" ("Motor References")) -> ("RobotDriveDevRef"=w218:T17)  [unwired: 9 in, 1 out]
    n136 = call <vilib>:"WPI_MotorControlRefNum Registry Get.vi"("refnum name"="Back Right Drive" ("Motor References")) -> ("RobotDriveDevRef"=w215:T17)  [unwired: 9 in, 1 out]
    n137 = call <vilib>:"Spark MAX Get Sensor Velocity.vi"("MotorControlDevRef in"=w218) -> ("Sensor Velocity"=→"Front Right RPM":dbl)  [unwired: 7 in, 3 out]
    n138 = call <vilib>:"Spark MAX Get Sensor Velocity.vi"("MotorControlDevRef in"=w215) -> ("Sensor Velocity"=→"Back Right RPM":dbl)  [unwired: 7 in, 3 out]
    n139 = Wait (ms)(milliseconds to wait=u32 100) -> ()  [unwired: 1 out]
  }
  n140 = while {
    stop <- FALSE stop-if-true
    # "Drive Commands Loop"
    n141 = global read "Robot Global Data.vi" "Robot Mode"() -> (w249:T9)
    n142 = global read "Robot Global Data.vi" "Robot Mode"() -> (w232:T9)
    n143 = Wait (ms)(milliseconds to wait=u32 30) -> ()  [unwired: 1 out]
    n144 = global read "Robot Global Data.vi" "Align 90"() -> (w246:bool)
    n145 = Equal?(x=WPI_DriverStationRobotMode2."Autonomous Enabled", y=w249) -> (x = y?=w247:bool)
    n146 = Equal?(x=WPI_DriverStationRobotMode2."Teleop Enabled", y=w232) -> (x = y?=w231:bool)
    n147 = And(x=w247, y=w246) -> (x .and. y?=w245:bool)
    n148 = And(x=w231, y="Align 90") -> (x .and. y?=w227:bool)
    n149 = Or(x=w245, y=w227) -> (x .or. y?=w228:bool)
    n150 = global read "Robot Global Data.vi" "Direction Commands"() -> (w252:T31)
    n151 = global read "Robot Global Data.vi" "Drive Commands"() -> (w253:T32)
    n152 = global read "Robot Global Data.vi" "Wheel Base Length"() -> (w251:dbl)
    n153 = global read "Robot Global Data.vi" "Wheel Base Width"() -> (w250:dbl)
    n154 = call <vilib>:"Swerve Drive Brushless V2.vi"("Front Left Offset"="Front Left Offset", "Direction"=w252, "Front Right Offset"="Front Right Offset", "Align 90"=w228, "Back Left  Offset"="Back Left Offset", "Wheel Base Length"=w251, "Back Right Offset"="Back Right Offset", "Drive Commands"=w253, "Wheel Base Width"=w250) -> ("Front Left Drive Output"=w244:T3, "Front Right Drive Output"=w241:T6, "Back Left Drive Output"=w243:T4, "Back Right Drive Output"=w242:T5)  [unwired: 3 in]
    "Left Front Drive Output" <- w244
    "Back Left Drive Output" <- w243
    "Back Right Drive Output" <- w242
    "Right  Front Drive Output" <- w241
    n155 = Unbundle By Name(w241) -> ("Front Right Current Angle"=w240:dbl)
    n156 = Unbundle By Name(w242) -> ("Back Right Current Angle"=w239:dbl)
    n157 = Unbundle By Name(w244) -> ("Front Left Current Angle"=w237:dbl)
    n158 = Unbundle By Name(w243) -> ("Back Left Current Angle"=w238:dbl)
    n159 = call-poly <vilib>:"NT Write Value.vi"("Numeric"=w237, "Name"="FL Angle") -> ()  [unwired: 9 in, 1 out]
    n160 = call-poly <vilib>:"NT Write Value.vi"("Numeric"=w238, "Name"="BL Angle") -> ()  [unwired: 9 in, 1 out]
    n161 = call-poly <vilib>:"NT Write Value.vi"("Numeric"=w239, "Name"="BR Angle") -> ()  [unwired: 9 in, 1 out]
    n162 = call-poly <vilib>:"NT Write Value.vi"("Numeric"=w240, "Name"="FR Angle") -> ()  [unwired: 9 in, 1 out]
  }
  n163 = while {
    stop <- FALSE stop-if-true
    # "Climber Commands Loop"
    n164 = Wait (ms)(milliseconds to wait=u32 30) -> ()  [unwired: 1 out]
    n165 = global read "Robot Global Data.vi" "Auxillary Axis"() -> (w329:T12)
    n166 = global read "Robot Global Data.vi" "Auxillary Buttons"() -> (w272:T13)
    n167 = global read "Robot Global Data.vi" "Auxillary POV"() -> (w271:cluster{"POV":i16})
    n168 = Unbundle By Name(w329) -> ("L Y Axis"=w303:dbl, "R Y Axis"=w298:dbl)
    n169 = Unbundle By Name(w271) -> ("POV"=w270:i16)
    n170 = Unbundle By Name(w272) -> ("Y"=w267:bool)
    n171 = Equal?(x=w270, y=i16 0) -> (x = y?=w268:bool)
    n172 = call <vilib>:"WPI_SwitchRefNum Registry Get.vi"("refnum name"=T10 "Rear Climber Limit Switch" ("Mechanisms")) -> ("error out"=w290:errorcluster, "SwitchDevRef"=w291:T34)  [unwired: 9 in]
    n173 = Or(x=w268, y=w267) -> (x .or. y?=w266:bool)
    n174 = call <vilib>:"WPI_SwitchRefNum Registry Get.vi"("refnum name"=T10 "Front Climber Limit Switch" ("Mechanisms")) -> ("error out"=w293:errorcluster, "SwitchDevRef"=w292:T34)  [unwired: 9 in]
    n175 = call "Toggle2.vi"("In 2"=w266) -> ("Out 2"=w306:bool)
    n176 = call <vilib>:"WPI_SwitchGetLimitValue.vi"("error in (no error)"=w290, "SwitchDevRef"=w291) -> ("Switch Pressed"=w286:bool)  [unwired: 7 in, 2 out]
    "Rear Climber Switch" <- w286
    n177 = call <vilib>:"WPI_SwitchGetLimitValue.vi"("error in (no error)"=w293, "SwitchDevRef"=w292) -> ("Switch Pressed"=w285:bool)  [unwired: 7 in, 2 out]
    "Front Climber Switch" <- w285
    n178 = call <vilib>:"WPI_SolenoidRefNum Registry Get.vi"("refnum name"=T10 "Front Claw" ("Mechanism")) -> ("error out"=w313:errorcluster, "SolenoidDevRef"=w312:T24)  [unwired: 9 in]
    n179 = Select(t=WPI_SolenoidValue."On" ("Value"), s=w306, f=WPI_SolenoidValue."Off" ("Value")) -> (s? t:f=w309:T22)
    n180 = call-poly <vilib>:"WPI_SolenoidSet.vi"("error in (no error)"=w313, "Value"=w309, "SolenoidDevRef"=w312) -> ("error out"=w310:errorcluster, "SolenoidDevRef"=w311:T24)  [unwired: 7 in]
    n181 = Not(x=w286) -> (.not. x?=w262:bool)
    n182 = call-poly <vilib>:"WPI_SolenoidGet.vi"("error in (no error)"=w310, "SolenoidDevRef"=w311) -> ("Value"=→"Claw Piston":bool)  [unwired: 7 in, 2 out]
    n183 = Not(x=w285) -> (.not. x?=w265:bool)
    n184 = Greater?(x=w298, y=0.75) -> (0:w261:bool)
    n185 = Less?(x=w298, y=-0.75) -> (x < y?=w284:bool)
    n186 = And(x=w262, y=w261) -> (x .and. y?=w260:bool)
    n187 = Greater?(x=w303, y=0.75) -> (0:w264:bool)
    n188 = Less?(x=w303, y=-0.75) -> (x < y?=w283:bool)
    n189 = And(x=w265, y=w264) -> (x .and. y?=w263:bool)
    n190 = call <vilib>:"WPI_MotorControlRefNum Registry Get.vi"("refnum name"=T10 "Rear Climber" ("Mechanism")) -> ("RobotDriveDevRef"=w322:T17)  [unwired: 9 in, 1 out]
    n191 = call <vilib>:"WPI_MotorControlRefNum Registry Get.vi"("refnum name"=T10 "Front Climber" ("Mechanism")) -> ("RobotDriveDevRef"=w315:T17)  [unwired: 9 in, 1 out]
    n192 = call <vilib>:"Spark MAX Get Sensor Position.vi"("MotorControlDevRef in"=w315) -> ("Sensor Position"=w274:dbl, "MotorControlDevRef out"=w314:T17)  [unwired: 7 in, 2 out]
    "Front Climber Postion" <- w274
    n193 = Greater?(x=w274, y="Front Stop") -> (0:w281:bool)
    n194 = And(x=w281, y=w283) -> (x .and. y?=w282:bool)
    n195 = Select(t=0.75, s=w260, f=0.0) -> (s? t:f=w327:dbl)
    n196 = call <vilib>:"Spark MAX Get Sensor Position.vi"("MotorControlDevRef in"=w322) -> ("Sensor Position"=w273:dbl, "MotorControlDevRef out"=w289:T17)  [unwired: 7 in, 2 out]
    "Rear Climber Postion" <- w273
    n197 = Greater?(x=w273, y="Rear Stop") -> (0:w278:bool)
    n198 = And(x=w278, y=w284) -> (x .and. y?=w279:bool)
    n199 = Select(t=-1.0, s=w279, f=w327) -> (s? t:f=w324:dbl)
    n200 = Select(t=1.0, s=w263, f=0.0) -> (s? t:f=w320:dbl)
    n201 = Select(t=-1.0, s=w282, f=w320) -> (s? t:f=w317:dbl)
    n202 = call <vilib>:"Spark MAX Set Output Advanced.vi"("Control Mode"=Spark_MAX_Control_Type."Percent VBus", "Setpoint"=w317, "MotorControlDevRef"=w314) -> ("MotorControlDevRef"=w288:T17)  [unwired: 7 in, 1 out]
    n203 = call <vilib>:"Spark MAX Set Output Advanced.vi"("Control Mode"=Spark_MAX_Control_Type."Percent VBus", "Setpoint"=w324, "MotorControlDevRef"=w289) -> ("MotorControlDevRef"=w287:T17)  [unwired: 7 in, 1 out]
    n204 = call-poly <vilib>:"NT Write Value.vi"("Numeric"=w273, "Name"="Rear Climber Postion") -> ()  [unwired: 9 in, 1 out]
    n205 = call-poly <vilib>:"NT Write Value.vi"("Numeric"=w274, "Name"="Front Climber Postion") -> ()  [unwired: 9 in, 1 out]
    n206 = case shown="True" w285 {
      tunnel: w288 -> [_ w334]
      frame False {
      }
      frame True {
        n207 = call <vilib>:"Spark MAX Set Sensor Position.vi"("Position"=0.0, "MotorControlDeviceRef"=w334) -> ()  [unwired: 8 in, 2 out]
      }
    }
    n208 = case shown="True" w286 {
      tunnel: w287 -> [_ w332]
      frame False {
      }
      frame True {
        n209 = call <vilib>:"Spark MAX Set Sensor Position.vi"("Position"=0.0, "MotorControlDeviceRef"=w332) -> ()  [unwired: 8 in, 2 out]
      }
    }
  }
  n210 = while {
    stop <- FALSE stop-if-true
    # "Shooter Commands Loop"
    n211 = Wait (ms)(milliseconds to wait=u32 30) -> ()  [unwired: 1 out]
    n212 = global read "Robot Global Data.vi" "Robot Mode"() -> (w349:T9)
    n213 = global read "Robot Global Data.vi" "Auto Shot Right"() -> (w346:bool)
    n214 = global read "Robot Global Data.vi" "Auxillary Axis"() -> (w370:T12)
    n215 = global read "Robot Global Data.vi" "Auto Shot left"() -> (w345:bool)
    n216 = Unbundle By Name(w370) -> ("LT"=w369:dbl, "RT"=w368:dbl)
    n217 = Equal?(x=WPI_DriverStationRobotMode2."Teleop Enabled", y=w349) -> (x = y?=w347:bool)
    n218 = case shown="True" w347 {
      tunnel: w369 -> [_ w427]
      tunnel: w368 -> [_ w426]
      tunnel: [w421 w423] -> w342
      tunnel: [w420 w422] -> w344
      tunnel: w346 -> [w421 _]
      tunnel: w345 -> [w420 _]
      frame False {
      }
      frame True {
        n219 = Greater?(x=w426, y=0.5) -> (0:w422:bool)
        n220 = Greater?(x=w427, y=0.5) -> (0:w423:bool)
      }
    }
    n221 = call "Pulse Switch.vi"("Input Switch"=w342, "Time/Loop Time"="Piston Delay") -> ("Pulse Switch"=w341:bool)  [unwired: 7 in, 1 out]
    n222 = call "Pulse Switch.vi"("Input Switch"=w344, "Time/Loop Time"="Piston Delay") -> ("Pulse Switch"=w343:bool)  [unwired: 7 in, 1 out]
    n223 = call <vilib>:"WPI_SolenoidRefNum Registry Get.vi"("refnum name"=T10 "Right Shooter Piston" ("Mechanism")) -> ("error out"=w367:errorcluster, "SolenoidDevRef"=w366:T24)  [unwired: 9 in]
    n224 = Select(t=WPI_SolenoidValue."On" ("Value"), s=w341, f=WPI_SolenoidValue."Off" ("Value")) -> (s? t:f=w363:T22)
    n225 = call-poly <vilib>:"WPI_SolenoidSet.vi"("error in (no error)"=w367, "Value"=w363, "SolenoidDevRef"=w366) -> ("error out"=w364:errorcluster, "SolenoidDevRef"=w365:T24)  [unwired: 7 in]
    n226 = call-poly <vilib>:"WPI_SolenoidGet.vi"("error in (no error)"=w364, "SolenoidDevRef"=w365) -> ("Value"=→"Right Shooter":bool)  [unwired: 7 in, 2 out]
    n227 = call <vilib>:"WPI_SolenoidRefNum Registry Get.vi"("refnum name"=T10 "Left Shooter Piston" ("Mechanism")) -> ("error out"=w358:errorcluster, "SolenoidDevRef"=w357:T24)  [unwired: 9 in]
    n228 = Select(t=WPI_SolenoidValue."On" ("Value"), s=w343, f=WPI_SolenoidValue."Off" ("Value")) -> (s? t:f=w354:T22)
    n229 = call-poly <vilib>:"WPI_SolenoidSet.vi"("error in (no error)"=w358, "Value"=w354, "SolenoidDevRef"=w357) -> ("error out"=w355:errorcluster, "SolenoidDevRef"=w356:T24)  [unwired: 7 in]
    n230 = global read "Robot Global Data.vi" "Robot Mode"() -> (w339:T9)
    n231 = global read "Robot Global Data.vi" "Auto Intake"() -> (w336:bool)
    n232 = call-poly <vilib>:"WPI_SolenoidGet.vi"("error in (no error)"=w355, "SolenoidDevRef"=w356) -> ("Value"=→"Left Shooter":bool)  [unwired: 7 in, 2 out]
    n233 = Equal?(x=WPI_DriverStationRobotMode2."Teleop Enabled", y=w339) -> (x = y?=w337:bool)
    n234 = case shown="True" w337 {
      tunnel: w336 -> [_ w403]
      frame True {
        n235 = global read "Robot Global Data.vi" "Auxillary POV"() -> (w395:cluster{"POV":i16})
        n236 = Unbundle(w395) -> ("POV"=w394:i16)
        n237 = Equal?(x=w394, y=i16 270) -> (x = y?=w396:bool)
        n238 = Equal?(x=i16 90, y=w394) -> (x = y?=w389:bool)
        n239 = call "Toggle2.vi"("In 2"=w396) -> ("Out 2"=w388:bool)
        n240 = call "Toggle2.vi"("In 2"=w389) -> ("Out 2"=w377:bool)
        n241 = Multiply(x=0.01, y="Low Goal") -> (x*y=w386:dbl)
        n242 = Select(t=w386, s=w388, f=0.0) -> (s? t:f=w374:dbl)
        n243 = Multiply(x=0.01, y="HIgh Left") -> (x*y=w375:dbl)
        n244 = Multiply(x=0.01, y="High Right") -> (x*y=w373:dbl)
        n245 = Select(t=w374, s=w377, f=w373) -> (s? t:f=w376:dbl)
        n246 = Select(t=w374, s=w377, f=w375) -> (s? t:f=w387:dbl)
        n247 = call <vilib>:"WPI_MotorControlRefNum Registry Get.vi"("refnum name"=T10 "Left Shooter Wheel" ("Mechanisms")) -> ("error out"=w382:errorcluster, "RobotDriveDevRef"=w381:T17)  [unwired: 9 in]
        n248 = call <vilib>:"WPI_MotorControlRefNum Registry Get.vi"("refnum name"=T10 "Right Shooter Wheel" ("Mechanisms")) -> ("error out"=w399:errorcluster, "RobotDriveDevRef"=w400:T17)  [unwired: 9 in]
        n249 = call <vilib>:"Spark MAX Set Output Advanced.vi"("error in (no error)"=w382, "Control Mode"=Spark_MAX_Control_Type."Percent VBus", "Setpoint"=w387, "MotorControlDevRef"=w381) -> ()  [unwired: 6 in, 2 out]
        n250 = call <vilib>:"Spark MAX Set Output Advanced.vi"("error in (no error)"=w399, "Control Mode"=Spark_MAX_Control_Type."Percent VBus", "Setpoint"=w376, "MotorControlDevRef"=w400) -> ()  [unwired: 6 in, 2 out]
      }
      frame False {
        w402 = 0.0 ("f")
        n251 = Multiply(x=0.01, y="HIgh Left 2") -> (x*y=w413:dbl)
        n252 = Multiply(x=0.01, y="High Right 2") -> (x*y=w405:dbl)
        n253 = Select(t=w413, s=w403, f=w402) -> (s? t:f=w414:dbl)
        n254 = Select(t=w405, s=w403, f=w402) -> (s? t:f=w404:dbl)
        n255 = call <vilib>:"WPI_MotorControlRefNum Registry Get.vi"("refnum name"=T10 "Left Shooter Wheel" ("Mechanisms")) -> ("error out"=w410:errorcluster, "RobotDriveDevRef"=w409:T17)  [unwired: 9 in]
        n256 = call <vilib>:"WPI_MotorControlRefNum Registry Get.vi"("refnum name"=T10 "Right Shooter Wheel" ("Mechanisms")) -> ("error out"=w417:errorcluster, "RobotDriveDevRef"=w418:T17)  [unwired: 9 in]
        n257 = call <vilib>:"Spark MAX Set Output Advanced.vi"("error in (no error)"=w410, "Control Mode"=Spark_MAX_Control_Type."Percent VBus", "Setpoint"=w414, "MotorControlDevRef"=w409) -> ()  [unwired: 6 in, 2 out]
        n258 = call <vilib>:"Spark MAX Set Output Advanced.vi"("error in (no error)"=w417, "Control Mode"=Spark_MAX_Control_Type."Percent VBus", "Setpoint"=w404, "MotorControlDevRef"=w418) -> ()  [unwired: 6 in, 2 out]
      }
    }
  }
  n259 = while {
    stop <- FALSE stop-if-true
    # "Teleop Control"
    n260 = global read "Robot Global Data.vi" "Robot Mode"() -> (w429:T9)
    n261 = Wait (ms)(milliseconds to wait=u32 30) -> ()  [unwired: 1 out]
    n262 = Equal?(x=WPI_DriverStationRobotMode2."Teleop Enabled", y=w429) -> (x = y?=w430:bool)
    n263 = case shown="True" w430 {
      frame False {
      }
      frame True {
        # "Switch front and back."
        n264 = global read "Robot Global Data.vi" "Driver Buttons"() -> (w455:T13)
        n265 = global read "Robot Global Data.vi" "Driver Axis"() -> (w449:T12)
        n266 = Unbundle By Name(w449) -> ("L X Axis"=w457:dbl, "L Y Axis"=w454:dbl, "R X Axis"=w456:dbl, "RT"=w450:dbl, "LT"=w448:dbl)
        n267 = Unbundle By Name(w455) -> ("LB"=w438:bool, "RB"=w437:bool, "Back"=w433:bool, "Start"=w436:bool)
        n268 = Greater?(x=w450, y=0.5) -> (0:w452:bool)
        n269 = Greater?(x=w448, y=0.5 ("f")) -> (0:w447:bool)
        n270 = call "Toggle2.vi"("In 2"=w452) -> ("Out 2"=w453:bool)
        n271 = global read "Robot Global Data.vi" "Drive Commands"() -> (w460:T32)
        n272 = Bundle By Name(cluster=w460, "Brake"=w447, "Coast"=w433, "Align Steer Motors"=w436, "Autonomous"=FALSE) -> (w458:T32)
        n273 = call "Toggle2.vi"("In 2"=w438) -> ("Out 2"=w435:bool)
        n274 = case shown="False" w453 {
          tunnel: [w523 w526] -> w467
          tunnel: w457 -> [w521 w526]
          tunnel: [w522 w525] -> w463
          tunnel: w454 -> [w520 w525]
          tunnel: [w519 w524] -> w465
          tunnel: w456 -> [w519 w524]
          frame False {
            n275 = Negate(x=w520) -> (-x=w522:dbl)
            n276 = Negate(x=w521) -> (-x=w523:dbl)
          }
          frame True {
          }
        }
        n277 = call "Toggle2.vi"("In 2"=w437) -> ("Out 2"=w434:bool)
        n278 = global write "Robot Global Data.vi" "Drive Commands"(w458) -> ()
        n279 = Negate(x=w467) -> (-x=w461:dbl)
        n280 = call "DeadBand.vi"("Deadband"=0.07, "Input"=w461) -> ("Output"=w441:dbl)  [unwired: 9 in]
        n281 = call "DeadBand.vi"("Deadband"=0.07, "Input"=w463) -> ("Output"=w440:dbl)  [unwired: 9 in]
        n282 = call "DeadBand.vi"("Deadband"=0.07, "Input"=w465) -> ("Output"=w439:dbl)  [unwired: 9 in]
        n283 = case shown="False" w434 {
          tunnel: w441 -> [w475 w500]
          tunnel: w440 -> [w474 w499]
          tunnel: w439 -> [w473 w498]
          tunnel: [w472 w497] -> w444
          tunnel: [w471 w496] -> w443
          tunnel: [w470 w495] -> w442
          tunnel: w435 -> [w469 w494]
          frame True {
            n284 = case shown="True" w469 {
              tunnel: [w483 w492] -> w472
              tunnel: [w482 w491] -> w471
              tunnel: [w481 w490] -> w470
              tunnel: w475 -> [w477 w488]
              tunnel: w474 -> [w478 w487]
              tunnel: w473 -> [w479 w486]
              frame True {
                w480 = 0.25 ("y")
                n285 = Multiply(x=w480, y=w478) -> (x*y=w482:dbl)
                n286 = Multiply(x=w480, y=w477) -> (x*y=w483:dbl)
                n287 = global write "Robot Global Data.vi" "Drive Speed Mode"("Slow" ("Drive Speed Mode")) -> ()
                n288 = Multiply(x=0.1 ("y"), y=w479) -> (x*y=w481:dbl)
              }
              frame False {
                w489 = 1.0 ("y")
                n289 = global write "Robot Global Data.vi" "Drive Speed Mode"("Turbo" ("Drive Speed Mode")) -> ()
                n290 = Multiply(x=w489, y=w487) -> (x*y=w491:dbl)
                n291 = Multiply(x=w489, y=w488) -> (x*y=w492:dbl)
                n292 = Multiply(x=0.4 ("y"), y=w486) -> (x*y=w490:dbl)
              }
            }
          }
          frame False {
            n293 = case shown="False" w494 {
              tunnel: [w508 w517] -> w497
              tunnel: [w507 w516] -> w496
              tunnel: [w506 w515] -> w495
              tunnel: w500 -> [w502 w513]
              tunnel: w499 -> [w503 w512]
              tunnel: w498 -> [w504 w511]
              frame True {
                w505 = 0.15 ("y")
                n294 = Multiply(x=w505, y=w503) -> (x*y=w507:dbl)
                n295 = Multiply(x=w505, y=w502) -> (x*y=w508:dbl)
                n296 = global write "Robot Global Data.vi" "Drive Speed Mode"("Slow" ("Drive Speed Mode")) -> ()
                n297 = Multiply(x=0.1 ("y"), y=w504) -> (x*y=w506:dbl)
              }
              frame False {
                w514 = 0.45 ("y")
                n298 = Multiply(x=w514, y=w512) -> (x*y=w516:dbl)
                n299 = Multiply(x=w514, y=w513) -> (x*y=w517:dbl)
                n300 = global write "Robot Global Data.vi" "Drive Speed Mode"("Normal" ("Drive Speed Mode")) -> ()
                n301 = Multiply(x=0.3 ("y"), y=w511) -> (x*y=w515:dbl)
              }
            }
          }
        }
        n302 = global read "Robot Global Data.vi" "Direction Commands"() -> (w445:T31)
        n303 = Bundle By Name(cluster=w445, "Lateral - X"=w444, "Longitudinal - Y"=w443, "Rotational - Z"=w442) -> (w446:T31)
        n304 = global write "Robot Global Data.vi" "Direction Commands"(w446) -> ()
      }
    }
  }
